vi "AddServo.vi"(8 "error in":errorcluster, 11 "Data in":T1) -> (0 "error out":errorcluster, 3 "Data out":T1)   [LabVIEW 2023]
uses:
  controls/UI Data.ctl
  <vilib>/Utility/miscctls.llb/LVStringsAndValuesArrayTypeDef_U16.ctl
  controls/ServoData.ctl
panel:
  out "Info":string
  in  "Cancel Button":bool
  in  "Channel":u16(ring) items=["0", "1", "2", "3", "4", "5"]
  in  "Confirm":bool
  in  "Name":string
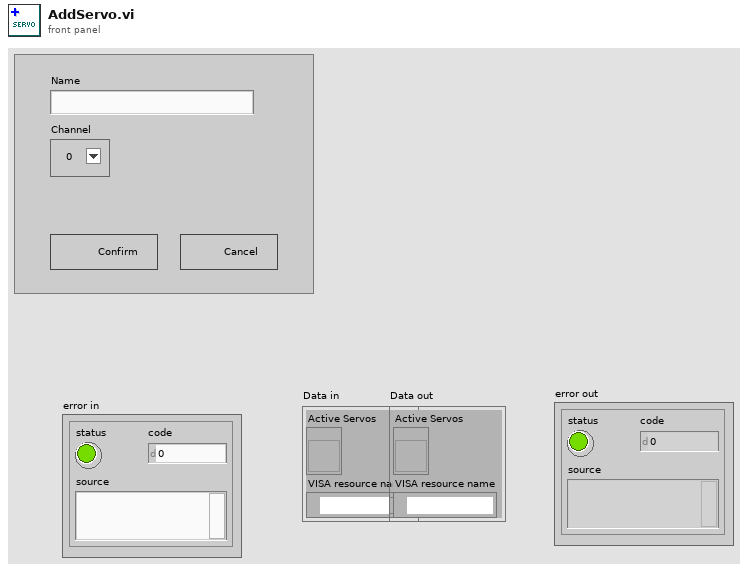
[diagram p1: front panel]
types:
  T1 = typedef "UI Data.ctl" = cluster{"Active Servos":refnum<vi>, "VISA resource name":refnum<visa-resource-name>}
  T2 = typedef "LVStringsAndValuesArrayTypeDef_U16.ctl" = cluster{"String":string, "Value":u16}[]
  T3 = typedef "ServoData.ctl" = cluster{"Name":string, "Channel":u8, "Delete Button":bool}
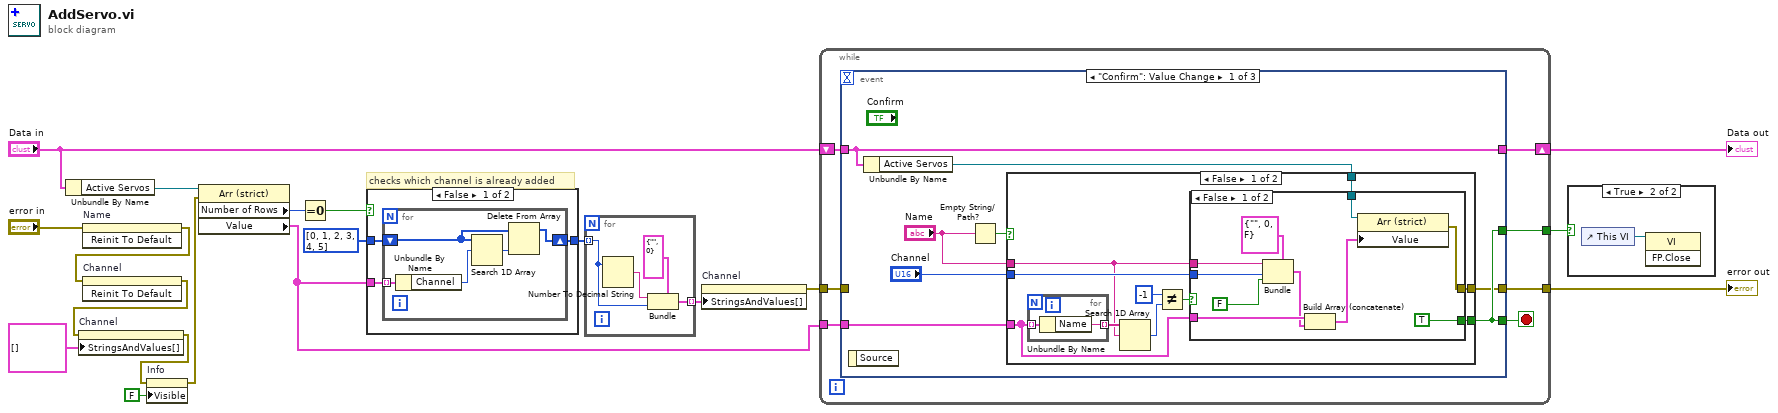
[diagram p0: block diagram]
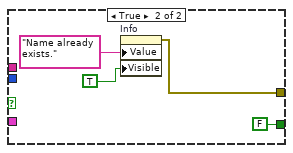
[diagram p3: hidden frame]
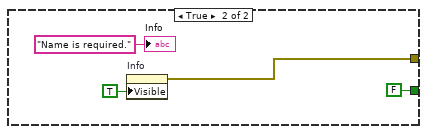
[diagram p4: hidden frame]
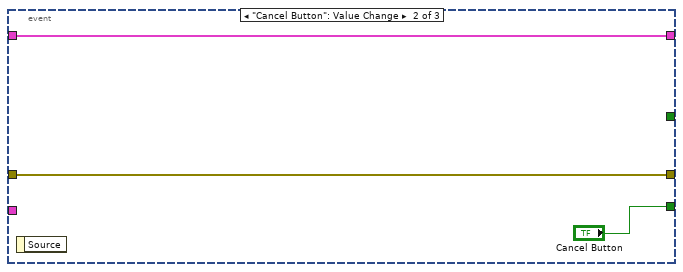
[diagram p5: hidden frame]
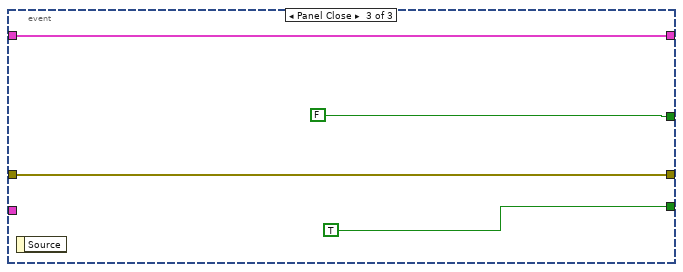
[diagram p6: hidden frame]
diagram:
  # "checks which channel is already added"
  n1 = Unbundle By Name("Data in") -> ("Active Servos"=w17:refnum<vi>)
  n2 = invoke on="Name" class="Str" method="Reinit To Default"(error in="error in") -> (error out=w9:errorcluster)  [unwired: 2 in, 2 out]
  n3 = invoke on="Channel" class="Ring (strict)" method="Reinit To Default"(error in=w9) -> (error out=w8:errorcluster)  [unwired: 2 in, 2 out]
  n4 = property on="Channel" class="Ring (strict)"(error in=w8, "StringsAndValues[]"=T2 [] ("Strings And Values []")) -> (error out=w2:errorcluster)  [unwired: 1 in, 1 out]
  n5 = property on="Info" class="Str"(error in=w2, "Visible"=FALSE) -> (error out=w1:errorcluster)  [unwired: 1 in, 1 out]
  n6 = property class="Arr (strict)"(reference=w17, error in=w1) -> ("Number of Rows"=w13:u32, "Value"=w6:T3[])  [unwired: 2 out]
  n7 = Equal To 0?(x=w13) -> (x = 0?=w12:bool)
  n8 = case shown="False" w12 {
    tunnel: w6 -> [w22 _]
    tunnel: u8[] [0, 1, 2, 3, 4, 5] -> [w21 w28]
    tunnel: [w20 w28] -> w15
    frame False {
      n9 = for {
        tunnel: w22 -> [w27] mode=indexing
        shift-right: [w23] -> w20
        shift-left: w21 -> [w25]
        n10 = Unbundle By Name(w27) -> ("Channel"=w26:u8)
        n11 = Search 1D Array(1D array=w25, element=w26) -> (index of element=w24:i32)  [unwired: 1 in]
        n12 = Delete From Array(array=w25, index=w24) -> (array with subset deleted=w23:u8[])  [unwired: 1 in, 1 out]
      }
    }
    frame True {
    }
  }
  n13 = for {
    tunnel: w15 -> [w31] mode=indexing
    tunnel: [w29] -> w14 mode=indexing
    n14 = Number To Decimal String(number=w31) -> (decimal integer string=w30:string)  [unwired: 1 in]
    n15 = Bundle(cluster=cluster{string, u16} {"", 0}, w30, w31) -> (w29:cluster{string, u16})
  }
  n16 = property on="Channel" class="Ring (strict)"("StringsAndValues[]"=w14) -> (error out=w11:errorcluster)  [unwired: 2 in, 1 out]
  n17 = while {
    shift-right: [w39] -> w19
    shift-left: "Data in" -> [w38]
    tunnel: w6 -> [w36]
    tunnel: w11 -> [w35]
    tunnel: [w34] -> w5
    tunnel: [w33] -> w4
    stop <- w37 stop-if-true
    n18 = event shown="[0] \"Confirm\": Value Change" {
      selector: _ -> [_ _ _]
      dyn-events: _ -> [_ _ _]
      timeout: _ -> [_ _ _]
      tunnel: [w46 w79 w83] -> w39
      tunnel: w38 -> [w46 w79 w83]
      tunnel: [w42 "Cancel Button" TRUE ("Cancel Button")] -> w37
      tunnel: w36 -> [w47 _ _]
      tunnel: w35 -> [_ w78 w82]
      tunnel: [w40 w78 w82] -> w34
      tunnel: [w42 _ FALSE ("Cancel Button")] -> w33
      event "Confirm": Value Change {
        n19 = event-data() -> ()  [unwired: 1 in, 1 out]
        n20 = Unbundle By Name(w46) -> ("Active Servos"=w41:refnum<vi>)
        n21 = Empty String/Path?(string/path="Name") -> (empty?=w43:bool)
        n22 = case shown="False" w43 {
          tunnel: w47 -> [w54 _]
          tunnel: "Channel" -> [w57 _]
          tunnel: "Name" -> [w55 _]
          tunnel: [w48 FALSE ("Cancel Button")] -> w42
          tunnel: w41 -> [w50 _]
          tunnel: [w49 w75] -> w40
          frame False {
            n23 = for {
              tunnel: w54 -> [w59] mode=indexing
              tunnel: [w58] -> w56 mode=indexing
              n24 = Unbundle By Name(w59) -> ("Name"=w58:string)
            }
            n25 = Search 1D Array(1D array=w56, element=w55) -> (index of element=w53:i32)  [unwired: 1 in]
            n26 = Not Equal?(x=-1, y=w53) -> (x != y?=w51:bool)
            n27 = case shown="False" w51 {
              tunnel: w54 -> [w67 _]
              tunnel: w57 -> [w65 _]
              tunnel: w55 -> [w64 _]
              tunnel: w50 -> [w62 _]
              tunnel: [w61 w71] -> w49
              tunnel: [TRUE ("Cancel Button") FALSE ("Cancel Button")] -> w48
              frame False {
                n28 = Bundle(cluster=T3 {"Name"="", "Channel"=0, "Delete Button"=FALSE} ("Servo data"), "Name"=w64, "Channel"=w65, "Delete Button"=FALSE) -> (w66:T3)
                n29 = Build Array (concatenate)(w67, w66) -> (w63:T3[])
                n30 = property class="Arr (strict)"(reference=w62, "Value"=w63) -> (error out=w61:errorcluster)  [unwired: 1 in, 1 out]
              }
              frame True {
                n31 = property on="Info" class="Str"("Value"="Name already exists." ("Info"), "Visible"=TRUE) -> (error out=w71:errorcluster)  [unwired: 2 in, 1 out]
              }
            }
          }
          frame True {
            n32 = property on="Info" class="Str"("Visible"=TRUE) -> (error out=w75:errorcluster)  [unwired: 2 in, 1 out]
            "Info" <- "Name is required." ("Info")
          }
        }
      }
      event "Cancel Button": Value Change {
        n33 = event-data() -> ()  [unwired: 1 in, 1 out]
      }
      event Panel Close {
        n34 = event-data() -> ()  [unwired: 1 in, 1 out]
      }
    }
  }
  "Data out" <- w19
  "error out" <- w5
  n35 = case shown="True" w4 {
    frame False {
    }
    frame True {
      n36 = control-ref of="This VI"() -> (w85:refnum<vi>)
      n37 = invoke class="VI" method="FP.Close"(reference=w85) -> ()  [unwired: 2 in, 3 out]
    }
  }
